vi "GoToTargetPosition.vi"(0 "object in":refnum<class "GoToSkill.lvclass">, 2 "Robot":refnum<class "Robot.lvclass">, 5 "error in (no error)":errorcluster) -> (14 "object out":refnum<class "GoToSkill.lvclass">, 16 "Robot out":refnum<class "Robot.lvclass">, 19 "error out":errorcluster)   [LabVIEW 2023, in "GoToSkill.lvclass"]
uses:
  GoToSkill.lvclass
  Robot_class/Robot.lvclass
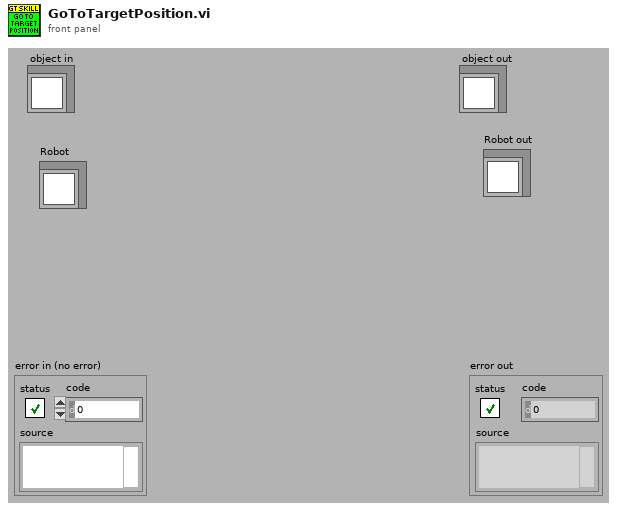
[diagram p1: front panel]
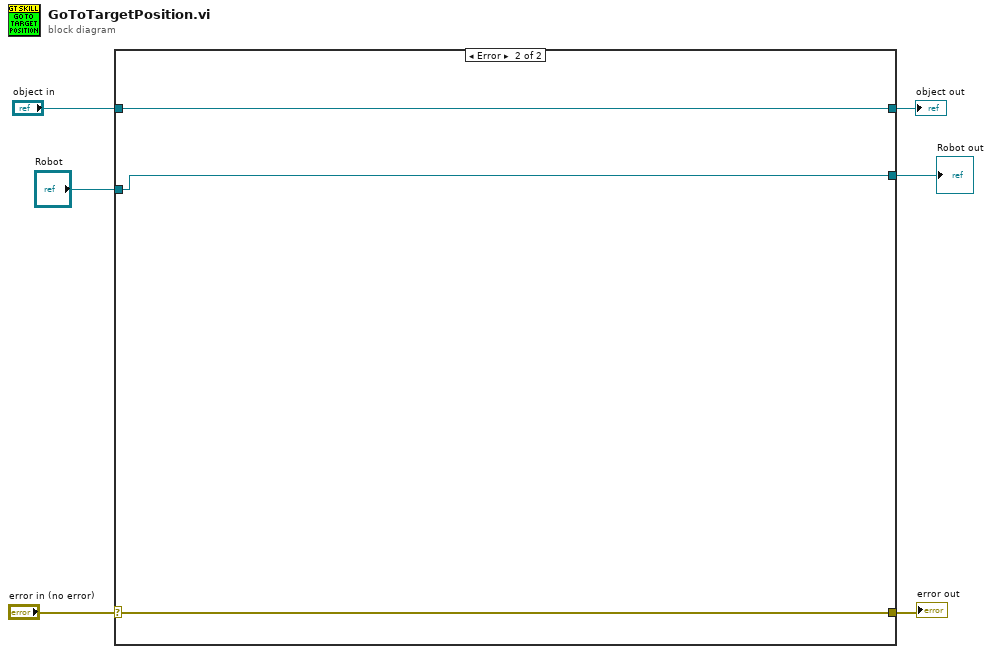
[diagram p0: block diagram]
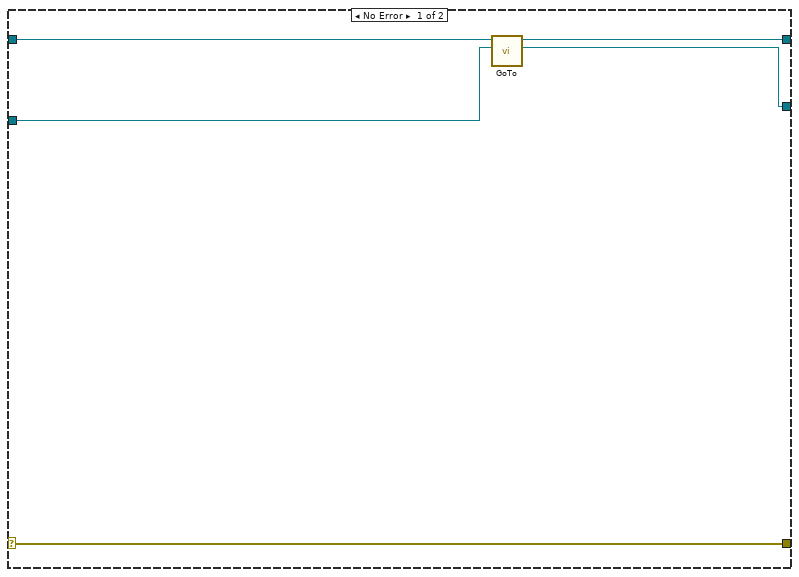
[diagram p2: hidden frame]
diagram:
  n1 = case shown="Error" "error in (no error)" {
    selector: "error in (no error)" -> [w11 w14]
    tunnel: [w11 w14] -> w5
    tunnel: [w9 w13] -> w3
    tunnel: "object in" -> [w10 w13]
    tunnel: "Robot" -> [w8 w12]
    tunnel: [w7 w12] -> w1
    frame No Error {
      n2 = call-dynamic "GoTo.vi"("Robot"=w8, "GoToSkill in"=w10) -> ("Robot out"=w7:refnum<class "Robot.lvclass">, "GoToSkill out"=w9:refnum<class "GoToSkill.lvclass">)  [unwired: 7 in, 1 out]
    }
    frame Error {
    }
  }
  "error out" <- w5
  "object out" <- w3
  "Robot out" <- w1
